vi "ZCAN_InitCAN(DTU).vi"(4 "error in (no error)":errorcluster caption="错误输入（无错误）", 5 "DTU系列初始化参数":T1, 6 "can_index":u32, 7 "device_hande":u32) -> (0 "error out":errorcluster caption="错误输出", 2 "can_index_handle":u32)   [LabVIEW 2018]
doc: "用于设置CAN通道的初始化参数。\n\n参数包括：波特率（自定义波特率）、工作模式；\n\n适用的设备：CANDTU-200XX, CANDTU-100UR"
uses:
  zlgcan_demo_CANFDNET_TCP/bin/zlgcan_wrap.dll
  data_type/ZCAN_InitCAN_setting_DTU.ctl
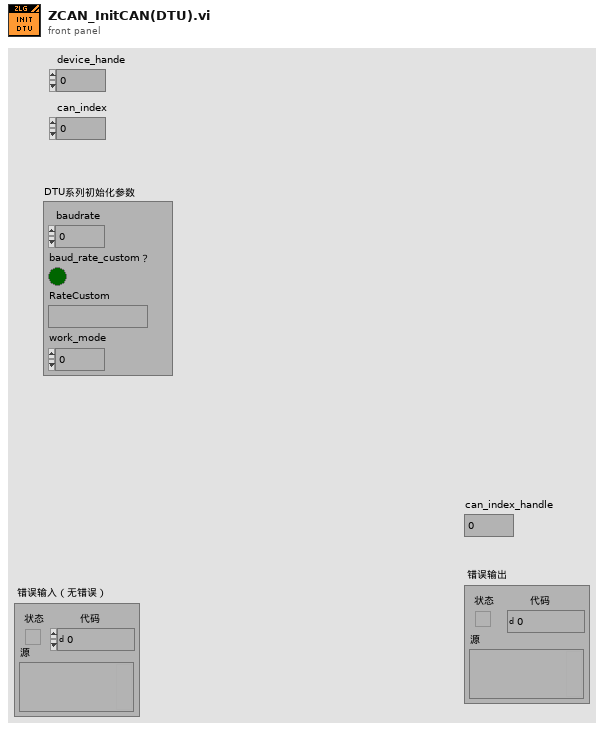
[diagram p1: front panel]
types:
  T1 = typedef "ZCAN_InitCAN_setting_DTU.ctl" = cluster{"baudrate":u32, "baud_rate_custom？":bool, "RateCustom":string, "work_mode":u32}
  T2 = cluster{"can_type":u32, "can_type":u32, "can_type":u32, "can_type":u32, "can_type":u8, "can_type":u8, "can_type":u8, "can_type":u8}
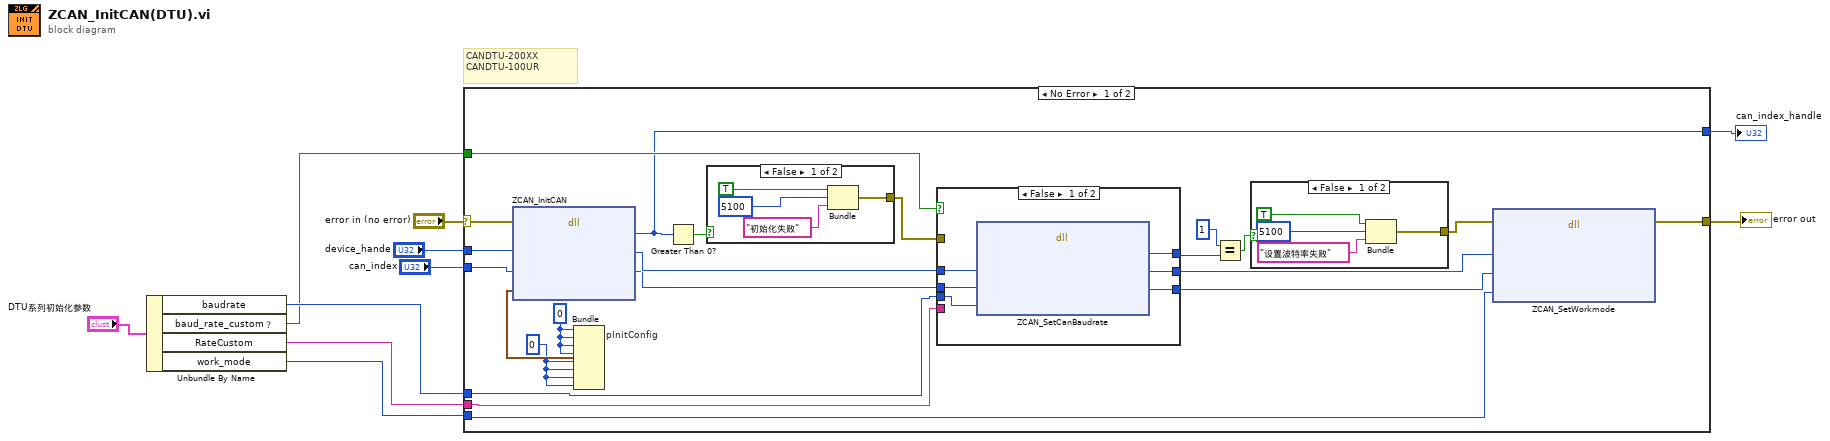
[diagram p0: block diagram]
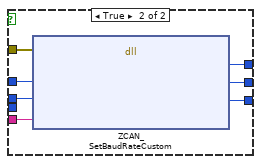
[diagram p3: hidden frame]
diagram:
  # "CANDTU-200XX\nCANDTU-100UR"
  n1 = Unbundle By Name("DTU系列初始化参数") -> ("baudrate"=w5:u32, "baud_rate_custom？"=w3:bool, "RateCustom"=w4:string, "work_mode"=w2:u32)
  n2 = case shown="No Error" "error in (no error)" {
    selector: "error in (no error)" -> [w26 _]
    tunnel: w3 -> [w17 _]
    tunnel: "device_hande" -> [w28 _]
    tunnel: "can_index" -> [w27 _]
    tunnel: w5 -> [w11 _]
    tunnel: [w12 _] -> w9
    tunnel: w4 -> [w16 _]
    tunnel: w2 -> [w30 _]
    tunnel: [w29 _] -> w1
    frame No Error {
      w25 = u8 0 ("can_type")
      w32 = u32 0 ("can_type")
      n3 = Bundle "pInitConfig"("can_type"=w32, "can_type"=w32, "can_type"=w32, "can_type"=w32, "can_type"=w25, "can_type"=w25, "can_type"=w25, "can_type"=w25) -> (w31:T2)  [unwired: 1 in]
      n4 = dll-call lib="C:/Users/admin/Desktop/zlgcan_demo_CANFDNET_TCP/bin/zlgcan_wrap.dll" fn="ZCAN_InitCAN"(error in=w26, "device_handle"=w28, "can_index"=w27, "pInitConfig"=w31) -> ("can_handle"=w12:u32, "device_handle"=w20:u32, "can_index"=w19:i32)  [unwired: 3 in, 2 out]
      n5 = Greater Than 0?(x=w12) -> (x > 0?=w24:bool)
      n6 = case shown="False" w24 {
        tunnel: [w50 _] -> w18
        frame False {
          n7 = Bundle("status"=TRUE, "code"=5100, "消息"="初始化失败") -> (w50:cluster{"status":bool, "code":i32, "消息":string})  [unwired: 1 in]
        }
        frame True {
        }
      }
      n8 = case shown="False" w17 {
        tunnel: w20 -> [w42 w49]
        tunnel: w19 -> [w41 w48]
        tunnel: [w39 w47] -> w14
        tunnel: [w38 w46] -> w13
        tunnel: w18 -> [_ w45]
        tunnel: [w40 w44] -> w23
        tunnel: w16 -> [_ w43]
        tunnel: w11 -> [w37 _]
        frame False {
          n9 = dll-call lib="C:/Users/admin/Desktop/zlgcan_demo_CANFDNET_TCP/bin/zlgcan_wrap.dll" fn="ZCAN_SetCanBaudrate"("hDev"=w42, "can_index"=w41, "baudrate"=w37) -> ("return"=w40:u32, "hDev"=w39:u32, "can_index"=w38:u32)  [unwired: 4 in, 2 out]
        }
        frame True {
          n10 = dll-call lib="C:/Users/admin/Desktop/zlgcan_demo_CANFDNET_TCP/bin/zlgcan_wrap.dll" fn="ZCAN_SetBaudRateCustom"(error in=w45, "device_handle"=w49, "can_index"=w48, "RateCustom"=w43) -> ("return"=w44:u32, "device_handle"=w47:u32, "can_index"=w46:u32)  [unwired: 3 in, 2 out]
        }
      }
      n11 = Equal?(x=1, y=w23) -> (x = y?=w22:bool)
      n12 = case shown="False" w22 {
        tunnel: [w33 _] -> w15
        frame False {
          n13 = Bundle("status"=TRUE, "code"=5100, "消息"="设置波特率失败") -> (w33:cluster{"status":bool, "code":i32, "消息":string})  [unwired: 1 in]
        }
        frame True {
        }
      }
      n14 = dll-call lib="C:/Users/admin/Desktop/zlgcan_demo_CANFDNET_TCP/bin/zlgcan_wrap.dll" fn="ZCAN_SetWorkmode" ("ZCAN_InitCAN")(error in=w15, "device_handle"=w14, "can_index"=w13, "work_mode"=w30) -> (error out=w29:errorcluster)  [unwired: 6 in, 1 out]
    }
    frame Error {
    }
  }
  "error out" <- w1
  "can_index_handle" <- w9
